vi "progress.vi"() -> ()   [LabVIEW 2009]
uses:
  <vilib>/vision/NI_Vision_Development_Module.lvlib
panel:
  out "XY Graph":cluster{"array":sgl[], "array":sgl[]}[](graph)
  out "tracked info":sgl[][](array[numeric])
  in  "start frame":i32
  in  "video length frames":i32=185
  in  "calibration frame":u32=2
  out "horizontal velocity":dbl format="%#_2g"
  out "vertical velocity":dbl format="%#_2g"
  out "horizontal velocity":cluster{"array":sgl[], "array":sgl[]}(graph)
  out "vertical velocity":cluster{"array":sgl[], "array":sgl[]}(graph)
  out "Image Out 2":T1(plugin-control)
  out "Centroid":cluster{"X Centroid":sgl, "Y Centroid":sgl} {"Y Centroid" format="%.2f"; "X Centroid" format="%.2f"}
  in  "stop":bool
  in  "AVI Path":path=path "C:/Users/Aspire/Desktop/kokum/weightlifting/lift1.avi"
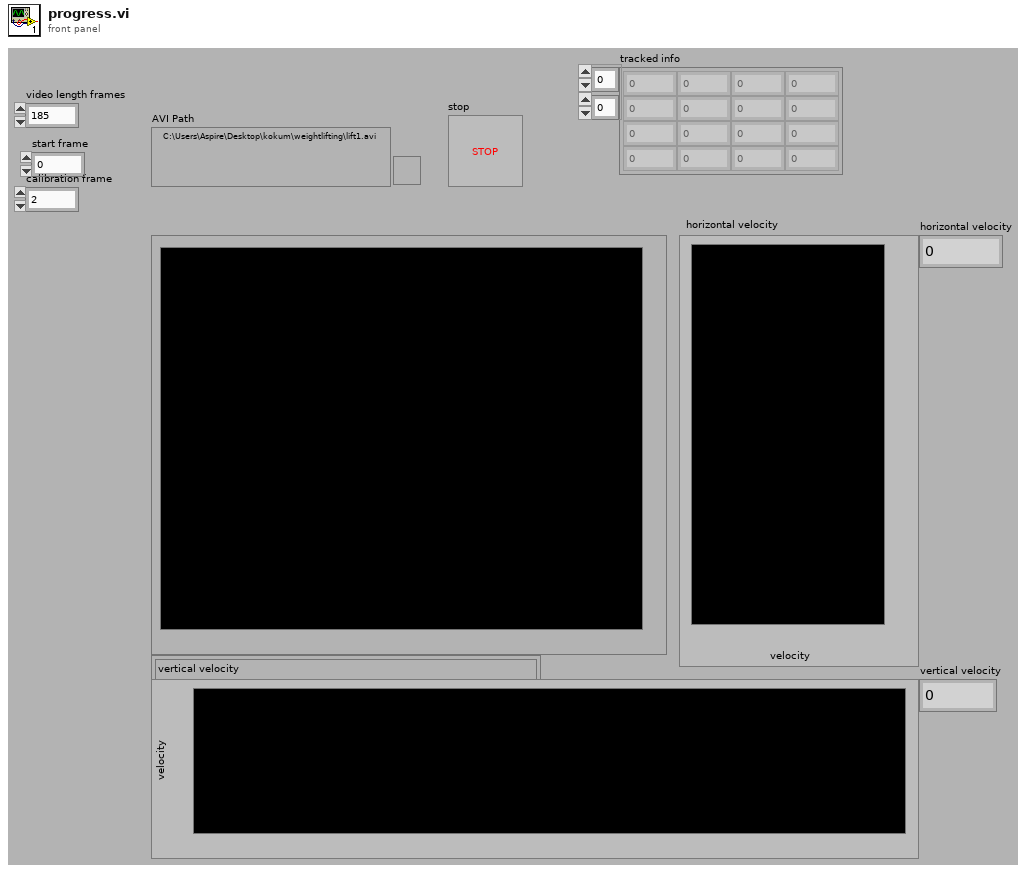
[diagram p1: front panel]
types:
  T1 = typedef "IMAQ Image.ctl" = refnum<image>
  T2 = typedef "AviRefnum.ctl" = refnum<k1>
  T3 = typedef "ROI Descriptor" = cluster{"Global Rectangle":i32[], "Contours":cluster{"ID":enum32{"External", "Internal"}, "Type":u32, "Coordinates":i32[]}[]}
  T4 = cluster{"ID":enum32{"External", "Internal"}, "Type":u32, "Coordinates":i32[]}[]
  T5 = cluster{"ID":enum32{"External", "Internal"}, "Type":u32, "Coordinates":i32[]}
  T6 = cluster{"ID":enum32{"External", "Internal"}, "Type":u32, dbl[]}
  T7 = cluster{"ID":enum32{"External", "Internal"}, "Type":u32, dbl[]}[]
  T8 = cluster{dbl[], cluster{"ID":enum32{"External", "Internal"}, "Type":u32, dbl[]}[]}
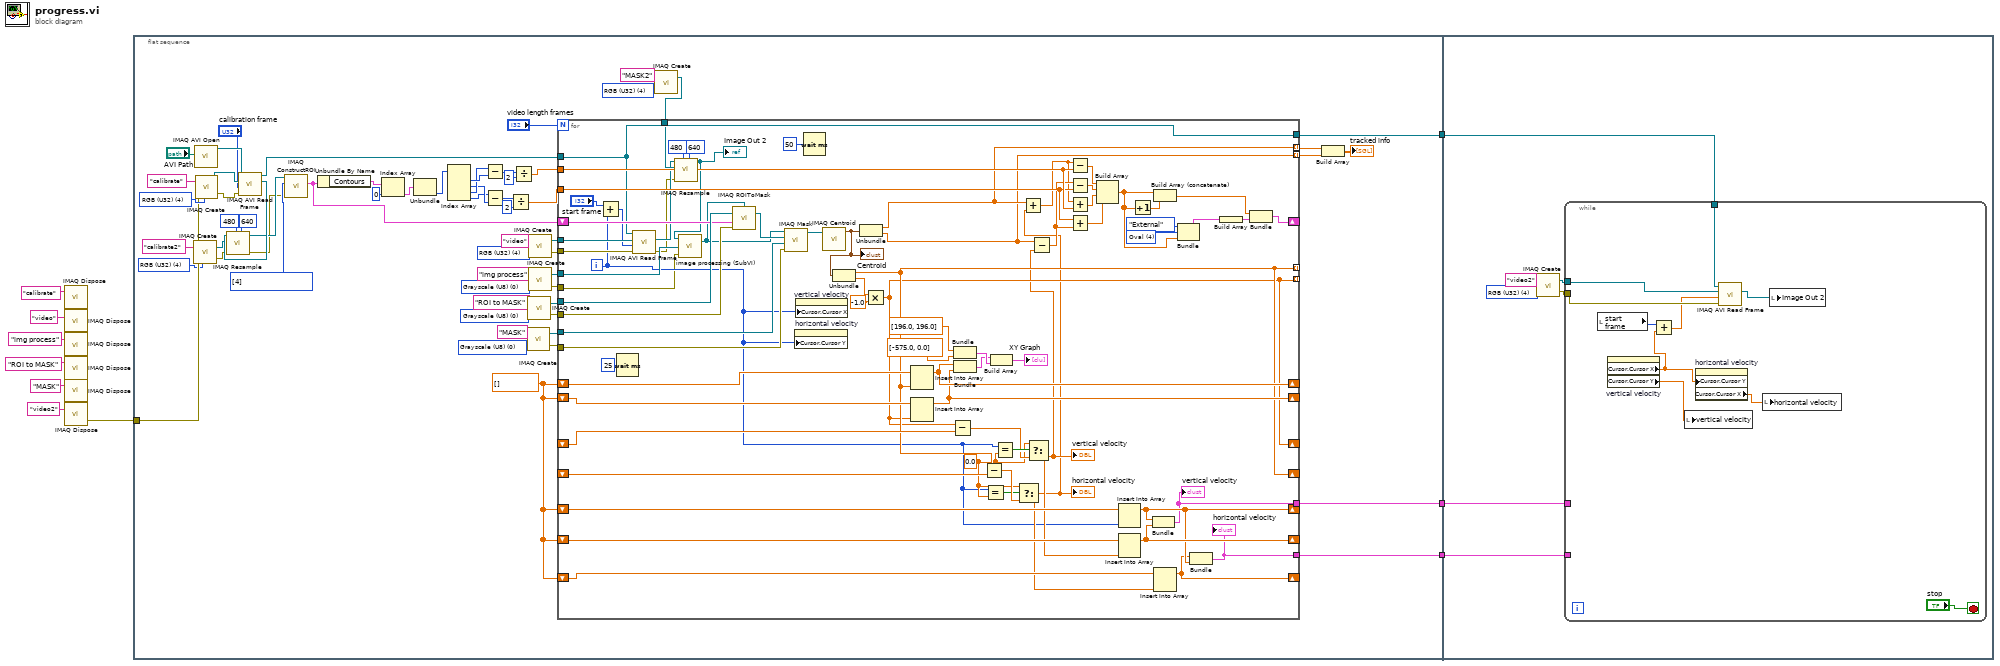
[diagram p0: block diagram]
diagram:
  n1 = call "IMAQ Dispose"("Image"="calibrate" ("Image Name")) -> ("error out"=w6:errorcluster)  [unwired: 5 in]
  n2 = call "IMAQ Dispose"("Image"="video" ("Image Name"), "error in (no error)"=w6) -> ("error out"=w5:errorcluster)  [unwired: 4 in]
  n3 = call "IMAQ Dispose"("Image"="img process" ("Image Name"), "error in (no error)"=w5) -> ("error out"=w4:errorcluster)  [unwired: 4 in]
  n4 = call "IMAQ Dispose"("Image"="ROI to MASK" ("Image Name"), "error in (no error)"=w4) -> ("error out"=w3:errorcluster)  [unwired: 4 in]
  n5 = call "IMAQ Dispose"("Image"="MASK" ("Image Name"), "error in (no error)"=w3) -> ("error out"=w2:errorcluster)  [unwired: 4 in]
  n6 = call "IMAQ Dispose"("Image"="video2" ("Image Name"), "error in (no error)"=w2) -> ("error out"=w1:errorcluster)  [unwired: 4 in]
  n7 = flat-sequence {
    tunnel: [w34] -> w15
    tunnel: [w33] -> w14
    tunnel: [w32] -> w13
    tunnel: w1 -> [w31]
    tunnel: w15 -> [w156]
    tunnel: w14 -> [w155]
    tunnel: w13 -> [w154]
    frame #0 {
      w17 = u32 4 items=["Grayscale (U8)", "Grayscale (I16)", "Grayscale (SGL)", "Complex (CSG)", "RGB (U32)", "HSL (U32)", "RGB (U64)"] ("Image Type")
      w22 = u32 4 items=["Grayscale (U8)", "Grayscale (I16)", "Grayscale (SGL)", "Complex (CSG)", "RGB (U32)", "HSL (U32)", "RGB (U64)"] ("Image Type")
      w35 = sgl[] [] ("array")
      w56 = u32[] [4] items=["No Selection", "Point", "Line", "Rectangle", "Oval", "Polygon", "Freehand Region", "Annulus", "Zoom", "Pan", "Broken Line", "Freehand Line", "Rotated Rectangle"] ("Tools")
      w64 = u32 4 items=["Grayscale (U8)", "Grayscale (I16)", "Grayscale (SGL)", "Complex (CSG)", "RGB (U32)", "HSL (U32)", "RGB (U64)"] ("Image Type")
      w66 = u32 0 items=["Grayscale (U8)", "Grayscale (I16)", "Grayscale (SGL)", "Complex (CSG)", "RGB (U32)", "HSL (U32)", "RGB (U64)"] ("Image Type")
      w68 = u32 0 items=["Grayscale (U8)", "Grayscale (I16)", "Grayscale (SGL)", "Complex (CSG)", "RGB (U32)", "HSL (U32)", "RGB (U64)"] ("Image Type")
      w71 = u32 0 items=["Grayscale (U8)", "Grayscale (I16)", "Grayscale (SGL)", "Complex (CSG)", "RGB (U32)", "HSL (U32)", "RGB (U64)"] ("Image Type")
      w75 = u32 4 items=["Grayscale (U8)", "Grayscale (I16)", "Grayscale (SGL)", "Complex (CSG)", "RGB (U32)", "HSL (U32)", "RGB (U64)"] ("Image Type")
      n8 = call "IMAQ Create"("Image Name"="calibrate2", "Image Type"=w22) -> ("New Image"=w21:T1, "error out"=w20:errorcluster)  [unwired: 3 in]
      n9 = call "IMAQ AVI Open"("AVI Path"="AVI Path") -> ("Avi Refnum"=w60:T2)  [unwired: 9 in, 1 out]
      n10 = call "IMAQ Create"("Image Name"="calibrate", "Image Type"=w64, "error in (no error)"=w31) -> ("New Image"=w62:T1, "error out"=w61:errorcluster)  [unwired: 2 in]
      n11 = call "IMAQ AVI Read Frame"("error in (no error)"=w61, "Frame Number"="calibration frame", "Image"=w62, "Avi Refnum"=w60) -> ("Image Out"=w25:T1, "Avi Refnum (duplicate)"=w37:T2)  [unwired: 4 in, 2 out]
      n12 = call "IMAQ Resample"("X Resolution"=640, "Y Resolution"=480, "error in (no error)"=w20, "Image Dst"=w21, "Image Src"=w25) -> ("error out"=w19:errorcluster, "Image Dst Out"=w24:T1)  [unwired: 5 in]
      n13 = call "IMAQ ConstructROI"("error in (no error)"=w19, "Tools"=w56, "Image"=w24) -> ("ROI Descriptor Out"=w46:T3)  [unwired: 5 in, 3 out]
      n14 = Unbundle By Name(w46) -> ("Contours"=w47:T4)
      n15 = Index Array(array=w47, index=0 ("Index")) -> (element=w48:T5)
      n16 = Unbundle(w48) -> ("Coordinates"=w45:i32[])  [unwired: 2 out]
      n17 = Index Array(array=w45) -> (element #1=w44:i32, element #2=w42:i32, element #3=w43:i32, element #4=w41:i32)  [unwired: 4 in]
      n18 = Subtract(x=w43, y=w44) -> (x-y=w55:i32)
      n19 = Subtract(x=w41, y=w42) -> (x-y=w53:i32)
      n20 = Divide(x=w53, y=2) -> (x/y=w50:dbl)
      n21 = Divide(x=w55, y=2) -> (x/y=w51:dbl)
      n22 = call "IMAQ Create"("Image Name"="MASK", "Image Type"=w66) -> ("New Image"=w59:T1, "error out"=w57:errorcluster)  [unwired: 3 in]
      n23 = call "IMAQ Create"("Image Name"="ROI to MASK", "Image Type"=w68) -> ("New Image"=w67:T1, "error out"=w58:errorcluster)  [unwired: 3 in]
      n24 = call "IMAQ Create"("Image Name"="video", "Image Type"=w75) -> ("New Image"=w73:T1, "error out"=w72:errorcluster)  [unwired: 3 in]
      n25 = call "IMAQ Create"("Image Name"="img process", "Image Type"=w71) -> ("New Image"=w39:T1, "error out"=w38:errorcluster)  [unwired: 3 in]
      n26 = call "IMAQ Create"("Image Name"="MASK2", "Image Type"=w17) -> ("New Image"=w16:T1)  [unwired: 3 in, 1 out]
      n27 = for {
        N: "video length frames" -> [_]
        tunnel: w73 -> [w149]
        tunnel: w72 -> [w148]
        tunnel: w37 -> [w97]
        tunnel: w67 -> [w147]
        tunnel: w59 -> [w146]
        tunnel: w58 -> [w144]
        tunnel: w57 -> [w145]
        shift-right: [w130] -> _
        shift-left: w46 -> [w142]
        tunnel: w51 -> [w141]
        tunnel: w50 -> [w140]
        tunnel: w39 -> [w129]
        tunnel: w38 -> [w82]
        shift-right: [w121] -> _
        shift-left: w35 -> [w123]
        shift-right: [w120] -> _
        shift-left: w35 -> [w122]
        shift-right: [w95] -> _
        shift-left: _ -> [w118]
        tunnel: [w107] -> _ mode=indexing
        tunnel: [w95] -> _ mode=indexing
        shift-right: [w107] -> _
        shift-left: _ -> [w108]
        shift-right: [w102] -> _
        shift-left: w35 -> [w106]
        shift-right: [w100] -> _
        shift-left: w35 -> [w104]
        shift-right: [w101] -> _
        shift-left: w35 -> [w105]
        tunnel: [w99] -> w33
        tunnel: [w98] -> w34
        tunnel: [w97] -> w32
        tunnel: [w85] -> w30 mode=indexing
        tunnel: [w84] -> w29 mode=indexing
        tunnel: w16 -> [w81]
        i -> [w89]
        w103 = 0.0 ("y")
        w133 = u32 4 items=["No Selection", "Point", "Line", "Rectangle", "Oval", "Polygon", "Free", "Annulus", "Unused2", "Unused3", "Broken Line", "Free Hand Line", "Rotated Rectangle"] ("Type")
        n28 = Add(x="start frame", y=w89) -> (x+y=w88:i32)
        n29 = Wait (ms)(milliseconds to wait=u32 25) -> ()  [unwired: 1 out]
        n30 = call "IMAQ AVI Read Frame"("error in (no error)"=w148, "Frame Number"=w88, "Image"=w149, "Avi Refnum"=w97) -> ("error out"=w78:errorcluster, "Image Out"=w80:T1)  [unwired: 4 in, 2 out]
        n31 = call "IMAQ Resample"("X Resolution"=640, "Y Resolution"=480, "error in (no error)"=w78, "Image Dst"=w81, "Image Src"=w80) -> ("Image Dst Out"=w79:T1)  [unwired: 5 in, 1 out]
        "Image Out 2" <- w79
        n32 = call "image processing (SubVI).vi"("error in"=w82, "Image dst"=w129, "Image src"=w79) -> ("Image Out"=w139:T1)  [unwired: 1 out]
        n33 = call "IMAQ ROIToMask"("error in (no error)"=w144, "ROI Descriptor"=w142, "Image"=w147, "Image Model"=w139) -> ("Image Out"=w143:T1)  [unwired: 2 in, 2 out]
        n34 = call "IMAQ Mask"("error in (no error)"=w145, "Image Dst"=w146, "Image Mask"=w143, "Image Src"=w139) -> ("Image Dst Out"=w138:T1)  [unwired: 1 in, 1 out]
        n35 = property on="horizontal velocity" class="XYGraph (strict)"("Cursor.Cursor Y"=w89) -> ()  [unwired: 2 in, 2 out]
        n36 = property on="vertical velocity" class="XYGraph (strict)"("Cursor.Cursor X"=w89) -> ()  [unwired: 2 in, 2 out]
        n37 = Wait (ms)(milliseconds to wait=u32 50) -> ()  [unwired: 1 out]
        n38 = call "IMAQ Centroid"("Image"=w138) -> ("Centroid"=w86:cluster{"X Centroid":sgl, "Y Centroid":sgl})  [unwired: 3 in, 1 out]
        "Centroid" <- w86
        n39 = Unbundle(w86) -> ("X Centroid"=w107:sgl, "Y Centroid"=w94:sgl)
        n40 = Unbundle(w86) -> ("X Centroid"=w85:sgl, "Y Centroid"=w84:sgl)
        n41 = Multiply(x=w94, y=-1.0) -> (x*y=w95:dbl)
        n42 = Insert Into Array(array=w123, new element=w107) -> (w121:sgl[])  [unwired: 1 in]
        n43 = Insert Into Array(array=w122, new element=w95) -> (w120:sgl[])  [unwired: 1 in]
        n44 = Subtract(x=w95, y=w118) -> (x-y=w117:dbl)
        n45 = Bundle("array"=sgl[] [196.0, 196.0], "array"=sgl[] [-575.0, 0.0]) -> (w114:cluster{"array":sgl[], "array":sgl[]})  [unwired: 1 in]
        n46 = Bundle("array"=w121, "array"=w120) -> (w113:cluster{"array":sgl[], "array":sgl[]})  [unwired: 1 in]
        n47 = Subtract(x=w107, y=w108) -> (x-y=w110:sgl)
        n48 = Equal?(x=w89, y=w103) -> (x = y?=w109:bool)
        n49 = Build Array(w113, w114) -> (→"XY Graph":cluster{"array":sgl[], "array":sgl[]}[])
        n50 = Equal?(x=w89, y=w103) -> (x = y?=w119:bool)
        n51 = Select(t=w103, s=w109, f=w110) -> (s? t:f=w91:dbl)
        "horizontal velocity" <- w91
        n52 = Add(x=w85, y=w91) -> (x+y=w90:dbl)
        n53 = Select(t=w103, s=w119, f=w117) -> (s? t:f=w93:dbl)
        "vertical velocity" <- w93
        n54 = Subtract(x=w84, y=w93) -> (x-y=w92:dbl)
        n55 = Subtract(x=w90, y=w141) -> (x-y=w127:dbl)
        n56 = Subtract(x=w92, y=w140) -> (x-y=w126:dbl)
        n57 = Add(x=w90, y=w141) -> (x+y=w125:dbl)
        n58 = Add(x=w140, y=w92) -> (x+y=w124:dbl)
        n59 = Build Array(w127, w126, w125, w124) -> (w128:dbl[])
        n60 = Insert Into Array(array=w105, new element=w89) -> (w101:sgl[])  [unwired: 1 in]
        n61 = Insert Into Array(array=w106, new element=w93) -> (w102:sgl[])  [unwired: 1 in]
        n62 = Increment(x=w128) -> (x+1=w132:dbl[])
        n63 = Bundle("array"=w101, "array"=w102) -> (w98:cluster{"array":sgl[], "array":sgl[]})  [unwired: 1 in]
        "vertical velocity" <- w98
        n64 = Build Array (concatenate)(w128, w132) -> (w131:dbl[])
        n65 = Insert Into Array(array=w104, new element=w91) -> (w100:sgl[])  [unwired: 1 in]
        n66 = Bundle("ID"=enum32{"External", "Internal"}."External", "Type"=w133, w128) -> (w135:T6)  [unwired: 1 in]
        n67 = Bundle("array"=w100, "array"=w101) -> (w99:cluster{"array":sgl[], "array":sgl[]})  [unwired: 1 in]
        "horizontal velocity" <- w99
        n68 = Build Array(w135) -> (w136:T7)
        n69 = Bundle(w131, w136) -> (w130:T8)  [unwired: 1 in]
      }
      n70 = Build Array(w30, w29) -> (→"tracked info":sgl[][])
    }
    frame #1 {
      w153 = u32 4 items=["Grayscale (U8)", "Grayscale (I16)", "Grayscale (SGL)", "Complex (CSG)", "RGB (U32)", "HSL (U32)", "RGB (U64)"] ("Image Type")
      n71 = call "IMAQ Create"("Image Name"="video2", "Image Type"=w153) -> ("New Image"=w151:T1, "error out"=w150:errorcluster)  [unwired: 3 in]
      n72 = while {
        tunnel: w156 -> [_]
        tunnel: w155 -> [_]
        tunnel: w154 -> [w165]
        tunnel: w151 -> [w164]
        tunnel: w150 -> [w163]
        stop <- "stop" stop-if-true
        n73 = local read "start frame"() -> (w159:i32)
        n74 = property on="vertical velocity" class="XYGraph (strict)"() -> ("Cursor.Cursor X"=w158:dbl, "Cursor.Cursor Y"=w161:dbl)  [unwired: 2 in, 2 out]
        n75 = Add(x=w159, y=w158) -> (x+y=w157:dbl)
        n76 = local write "vertical velocity"(w161) -> ()
        n77 = property on="horizontal velocity" class="XYGraph (strict)"("Cursor.Cursor Y"=w158) -> ("Cursor.Cursor X"=w160:dbl)  [unwired: 2 in, 2 out]
        n78 = call "IMAQ AVI Read Frame"("error in (no error)"=w163, "Frame Number"=w157, "Image"=w164, "Avi Refnum"=w165) -> ("Image Out"=w162:T1)  [unwired: 4 in, 3 out]
        n79 = local write "horizontal velocity"(w160) -> ()
        n80 = local write "Image Out 2"(w162) -> ()
      }
    }
  }
